vi "setUpShiftSpeeds.vi"(8 "error in (no error)":errorcluster, 11 "AndorIKonAcquisitor in":refnum<class "AndorIKonAcquisitor.lvclass">) -> (0 "error out":errorcluster, 3 "AndorIKonAcquisitor out":refnum<class "AndorIKonAcquisitor.lvclass">)   [LabVIEW 2009, in "Hardware.lvlib" / "Channels.lvlib" / "AndorIKonAcquisitor.lvclass"]
uses:
  AndorIKonAcquisitor.lvclass
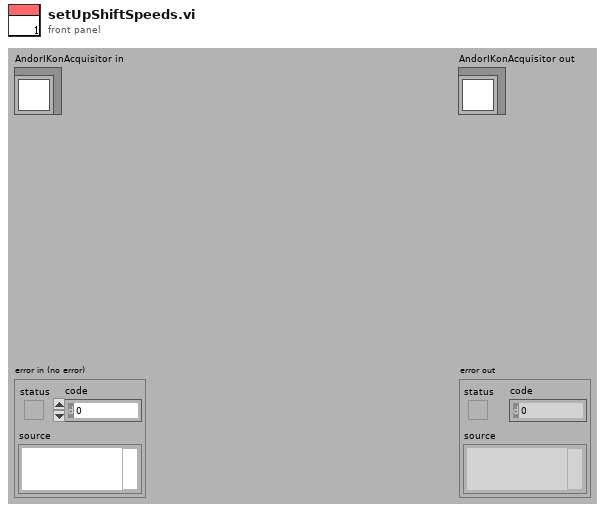
[diagram p1: front panel]
types:
  T1 = cluster{"Vertical Shift Speed":dbl, "Horizontal Shift Speed":dbl, "Fast Kinetic V Shift Speed":dbl}
  T2 = cluster{"Vertical Shift Speeds":dbl[], "Horizontal Shift Speeds":dbl[]}
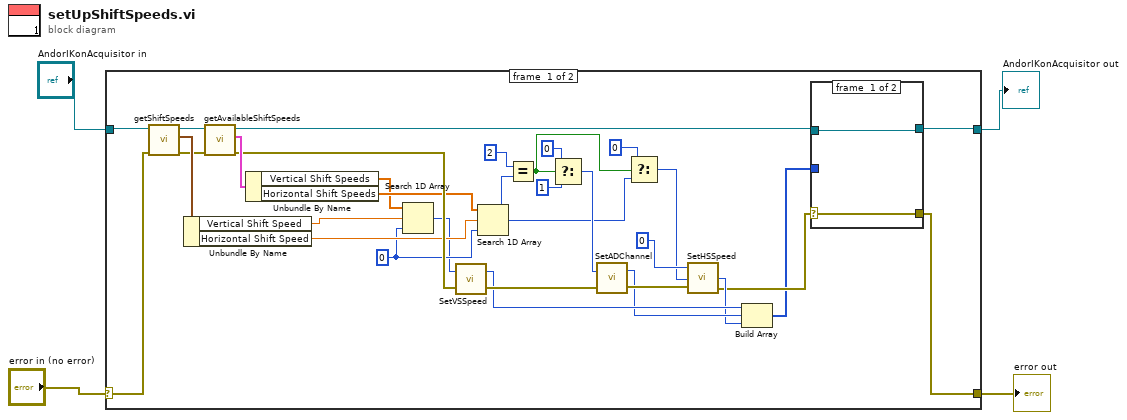
[diagram p0: block diagram]
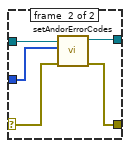
[diagram p2: hidden frame]
diagram:
  n1 = case shown="No Error" "error in (no error)" {
    selector: "error in (no error)" -> [w11 w45]
    tunnel: [w7 w45] -> w3
    tunnel: [w8 w44] -> w1
    tunnel: "AndorIKonAcquisitor in" -> [w12 w44]
    frame #0 {
      w19 = 0
      n2 = call-dynamic "getShiftSpeeds.vi"("error in (no error)"=w11, "CameraAcquisitor.lvclass in"=w12) -> ("error out"=w35:errorcluster, "Shift Speed"=w36:T1, "CameraAcquisitor.lvclass out"=w10:refnum<class "AndorIKonAcquisitor.lvclass">)  [unwired: 7 in]
      n3 = Unbundle By Name(w36) -> ("Vertical Shift Speed"=w33:dbl, "Horizontal Shift Speed"=w30:dbl)
      n4 = call "getAvailableShiftSpeeds.vi"("error in (no error)"=w35, "AndorIKonAcquisitor.lvclass in"=w10) -> ("error out"=w32:errorcluster, "Available Shift Speeds"=w34:T2, "AndorIKonAcquisitor.lvclass out"=w9:refnum<class "AndorIKonAcquisitor.lvclass">)  [unwired: 7 in]
      n5 = Unbundle By Name(w34) -> ("Vertical Shift Speeds"=w20:dbl[], "Horizontal Shift Speeds"=w31:dbl[])
      n6 = Search 1D Array(1D array=w20, element=w33, start index (0)=w19) -> (index of element=w18:i32)
      n7 = call <userlib>:"SetVSSpeed.vi"("error in (no error)"=w32, "index"=w18) -> ("error out"=w26:errorcluster, "DLL error code"=w23:u32)
      n8 = Search 1D Array(1D array=w31, element=w30, start index (0)=w19) -> (index of element=w14:i32)
      n9 = Equal?(x=2, y=w14) -> (x = y?=w17:bool)
      n10 = Select(t=0, s=w17, f=1) -> (s? t:f=w27:i32)
      n11 = call <userlib>:"SetADChannel.vi"("error in (no error)"=w26, "channel"=w27) -> ("error out"=w24:errorcluster, "DLL error code"=w22:u32)
      n12 = Select(t=0, s=w17, f=w14) -> (s? t:f=w13:i32)
      n13 = call <userlib>:"SetHSSpeed.vi"("error in (no error)"=w24, "index"=w13, "type"=0) -> ("error out"=w6:errorcluster, "DLL error code"=w21:u32)  [unwired: 1 in]
      n14 = Build Array(w23, w22, w21) -> (w5:u32[])
      n15 = case shown="Error" w6 {
        selector: w6 -> [w38 w43]
        tunnel: w9 -> [w37 w39]
        tunnel: [w37 w41] -> w8
        tunnel: [w38 w42] -> w7
        tunnel: w5 -> [_ w40]
        frame #0 {
        }
        frame #1 {
          n16 = call-dynamic "setAndorErrorCodes.vi"("error in (no error)"=w43, "Andor Error Codes"=w40, "AndorIKonAcquisitor.lvclass in"=w39) -> ("error out"=w42:errorcluster, "AndorIKonAcquisitor.lvclass out"=w41:refnum<class "AndorIKonAcquisitor.lvclass">)  [unwired: 7 in]
        }
      }
    }
    frame #1 {
    }
  }
  "error out" <- w3
  "AndorIKonAcquisitor out" <- w1
